vi "Test Sleep FTE.vi"() -> ()   [LabVIEW 2021]
uses:
  Time Conversion/LabVIEW Time to UTC Time.vi
  SubVIs/Add Error.vi
  CIFCore/Common/Utilities/Append Error Location.vi
  CIFClocks.lvlib
panel:
  out "Sleep Errors":i64[](array[numeric])
  out "status":string
  out "pass":bool
  out "error out":errorcluster
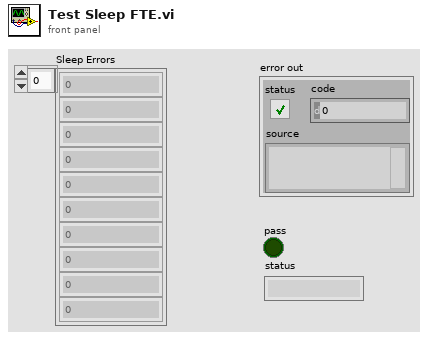
[diagram p1: front panel]
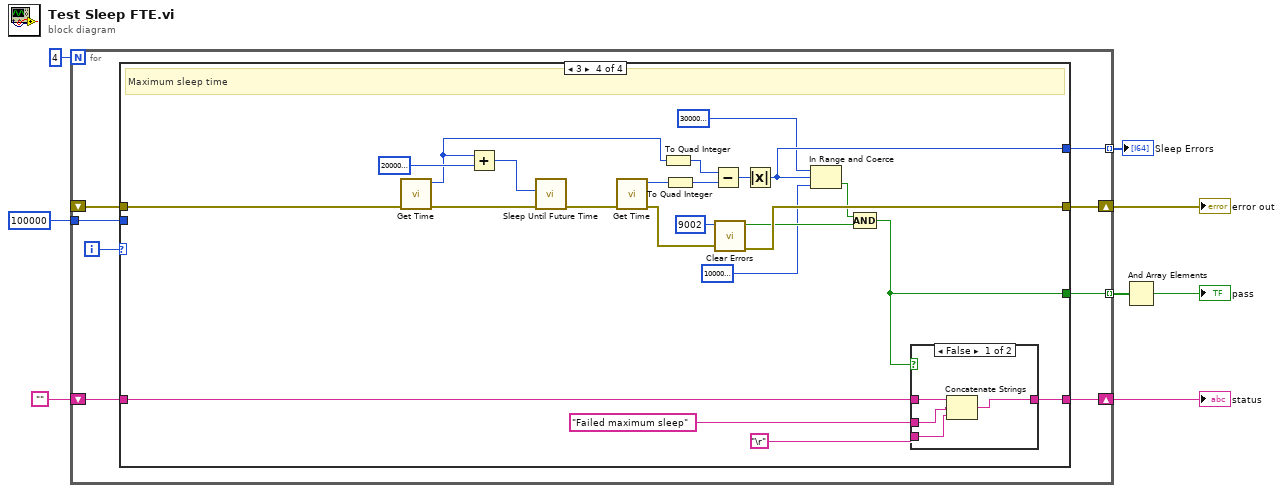
[diagram p0: block diagram]
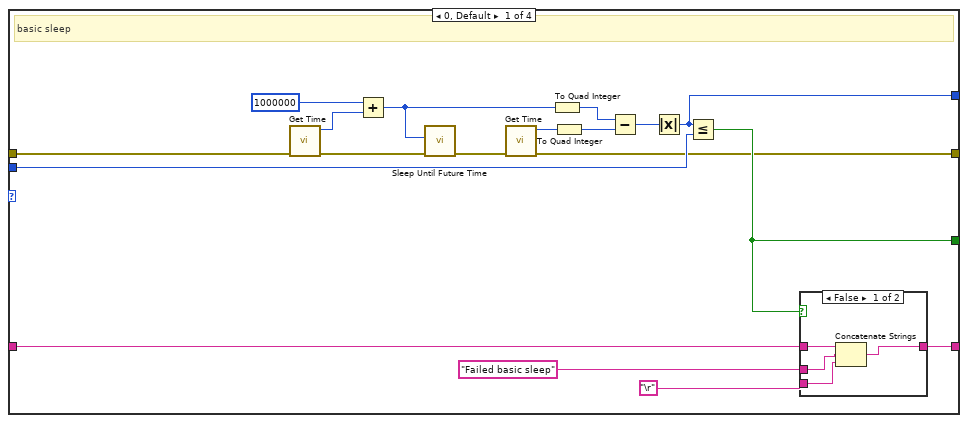
[diagram p2: hidden frame]
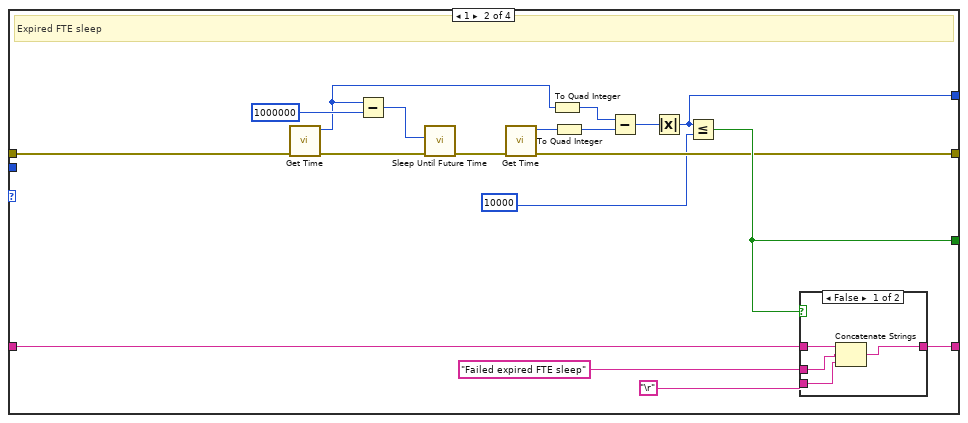
[diagram p4: hidden frame]
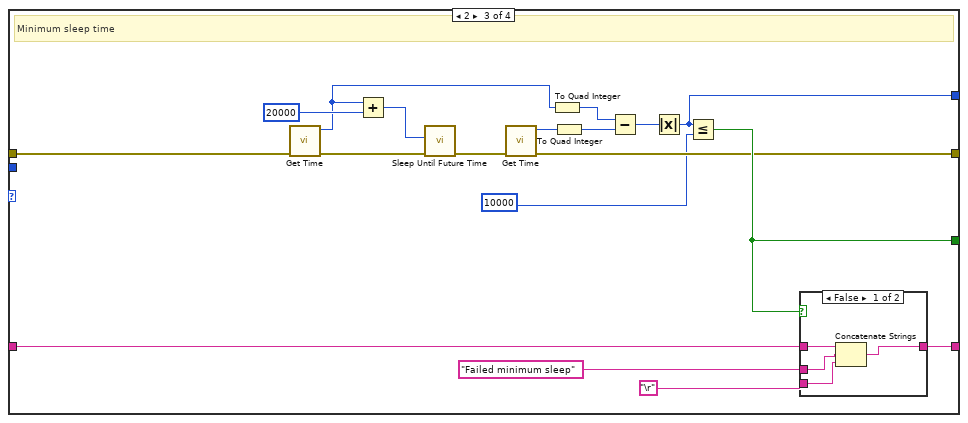
[diagram p6: hidden frame]
diagram:
  n1 = for {
    N: 4 -> [_]
    tunnel: [w16] -> w8 mode=indexing
    shift-right: [w13] -> w4
    shift-left: "" -> [w14]
    tunnel: i64 100000 ("y") -> [w12]
    shift-right: [w11] -> w2
    shift-left: _ -> [w10]
    tunnel: [w9] -> w1 mode=indexing
    i -> [w15]
    n2 = case shown="3" w15 {
      tunnel: [w20 w45 w68 w90] -> w16
      tunnel: w14 -> [w34 w57 w80 w108]
      tunnel: [w33 w56 w79 w107] -> w13
      tunnel: w12 -> [w21 _ _ _]
      tunnel: [w19 w44 w67 w92] -> w11
      tunnel: w10 -> [w18 w43 w66 w96]
      tunnel: [w17 w42 w65 w89] -> w9
      frame 0, Default {
        # "basic sleep"
        n3 = call "Get Time.vi"("error in (no error)"=w18) -> ("error out"=w29:errorcluster, "Time (ns)"=w30:u64)  [unwired: 8 in, 1 out]
        n4 = Add(x=u64 1000000, y=w30) -> (x+y=w26:u64)
        n5 = call "Sleep Until Future Time.vi"("error in (no error)"=w29, "Wake Time"=w26) -> ("error out"=w27:errorcluster)  [unwired: 9 in]
        n6 = call "Get Time.vi"("error in (no error)"=w27) -> ("error out"=w19:errorcluster, "Time (ns)"=w25:u64)  [unwired: 8 in, 1 out]
        n7 = To Quad Integer(1:w26) -> (0:w24:i64)
        n8 = To Quad Integer(1:w25) -> (0:w23:i64)
        n9 = Subtract(x=w24, y=w23) -> (x-y=w22:i64)
        n10 = Absolute Value(x=w22) -> (abs(x)=w17:i64)
        n11 = Less Or Equal?(x=w17, y=w21) -> (x <= y?=w20:bool)
        n12 = case shown="False" w20 {
          tunnel: w34 -> [w38 w39]
          tunnel: [w35 w39] -> w33
          tunnel: "Failed basic sleep" -> [w37 _]
          tunnel: "\r" -> [w36 _]
          frame False {
            n13 = Concatenate Strings(w38, w37, w36) -> (w35:string)
          }
          frame True {
          }
        }
      }
      frame 1 {
        # "Expired FTE sleep"
        n14 = call "Get Time.vi"("error in (no error)"=w43) -> ("error out"=w53:errorcluster, "Time (ns)"=w41:u64)  [unwired: 8 in, 1 out]
        n15 = Subtract(x=w41, y=u64 1000000 ("x")) -> (x-y=w50:u64)
        n16 = call "Sleep Until Future Time.vi"("error in (no error)"=w53, "Wake Time"=w50) -> ("error out"=w51:errorcluster)  [unwired: 9 in]
        n17 = call "Get Time.vi"("error in (no error)"=w51) -> ("error out"=w44:errorcluster, "Time (ns)"=w49:u64)  [unwired: 8 in, 1 out]
        n18 = To Quad Integer(1:w41) -> (0:w48:i64)
        n19 = To Quad Integer(1:w49) -> (0:w47:i64)
        n20 = Subtract(x=w48, y=w47) -> (x-y=w46:i64)
        n21 = Absolute Value(x=w46) -> (abs(x)=w42:i64)
        n22 = Less Or Equal?(x=w42, y=i64 10000) -> (x <= y?=w45:bool)
        n23 = case shown="False" w45 {
          tunnel: w57 -> [w61 w62]
          tunnel: [w58 w62] -> w56
          tunnel: "Failed expired FTE sleep" -> [w60 _]
          tunnel: "\r" -> [w59 _]
          frame False {
            n24 = Concatenate Strings(w61, w60, w59) -> (w58:string)
          }
          frame True {
          }
        }
      }
      frame 2 {
        # "Minimum sleep time"
        n25 = call "Get Time.vi"("error in (no error)"=w66) -> ("error out"=w76:errorcluster, "Time (ns)"=w64:u64)  [unwired: 8 in, 1 out]
        n26 = Add(x=w64, y=u64 20000 ("x")) -> (x+y=w73:u64)
        n27 = call "Sleep Until Future Time.vi"("error in (no error)"=w76, "Wake Time"=w73) -> ("error out"=w74:errorcluster)  [unwired: 9 in]
        n28 = call "Get Time.vi"("error in (no error)"=w74) -> ("error out"=w67:errorcluster, "Time (ns)"=w72:u64)  [unwired: 8 in, 1 out]
        n29 = To Quad Integer(1:w64) -> (0:w71:i64)
        n30 = To Quad Integer(1:w72) -> (0:w70:i64)
        n31 = Subtract(x=w71, y=w70) -> (x-y=w69:i64)
        n32 = Absolute Value(x=w69) -> (abs(x)=w65:i64)
        n33 = Less Or Equal?(x=w65, y=i64 10000) -> (x <= y?=w68:bool)
        n34 = case shown="False" w68 {
          tunnel: w80 -> [w84 w85]
          tunnel: [w81 w85] -> w79
          tunnel: "Failed minimum sleep" -> [w83 _]
          tunnel: "\r" -> [w82 _]
          frame False {
            n35 = Concatenate Strings(w84, w83, w82) -> (w81:string)
          }
          frame True {
          }
        }
      }
      frame 3 {
        # "Maximum sleep time"
        n36 = call "Get Time.vi"("error in (no error)"=w96) -> ("error out"=w104:errorcluster, "Time (ns)"=w95:u64)  [unwired: 8 in, 1 out]
        n37 = Add(x=w95, y=u64 2000000000 ("x")) -> (x+y=w101:u64)
        n38 = call "Sleep Until Future Time.vi"("error in (no error)"=w104, "Wake Time"=w101) -> ("error out"=w102:errorcluster)  [unwired: 9 in]
        n39 = call "Get Time.vi"("error in (no error)"=w102) -> ("error out"=w94:errorcluster, "Time (ns)"=w100:u64)  [unwired: 8 in, 1 out]
        n40 = To Quad Integer(1:w95) -> (0:w99:i64)
        n41 = To Quad Integer(1:w100) -> (0:w98:i64)
        n42 = Subtract(x=w99, y=w98) -> (x-y=w97:i64)
        n43 = call <vilib>:"Clear Errors.vi"("error in (no error)"=w94, "specific error code to clear (0: all)"=9002) -> ("error out"=w92:errorcluster, "specific error cleared?"=w91:bool)  [unwired: 4 in]
        n44 = Absolute Value(x=w97) -> (abs(x)=w89:i64)
        n45 = In Range and Coerce(upper limit=i64 300000000 ("y"), x=w89, lower limit=i64 100000000 ("y")) -> (In Range?=w88:bool)  [unwired: 1 out]
        n46 = Compound Arithmetic op=AND(w88, w91) -> (w90:bool)
        n47 = case shown="False" w90 {
          tunnel: w108 -> [w112 w113]
          tunnel: [w109 w113] -> w107
          tunnel: "Failed maximum sleep" -> [w111 _]
          tunnel: "\r" -> [w110 _]
          frame False {
            n48 = Concatenate Strings(w112, w111, w110) -> (w109:string)
          }
          frame True {
          }
        }
      }
    }
  }
  "error out" <- w2
  "status" <- w4
  "Sleep Errors" <- w1
  n49 = And Array Elements(Boolean array=w8) -> (logical AND=→"pass":bool)
